vi "Is OD Sub-Entry.vi"(8 "error in":errorcluster, 11 "Section Name in":refnum<class "Section Name.lvclass">) -> (0 "error out":errorcluster, 1 "Is OD Entry?":bool, 2 "Index":u16 format="%.0x", 3 "Section Name out":refnum<class "Section Name.lvclass">)   [LabVIEW 2020, in "Electronic Datasheet.lvlib" / "Section Name.lvclass"]
uses:
  Section Name.lvclass
  Section Name.lvclass/Section Name.ctl
  <vilib>/regexp/Match Regular Expression.xnode
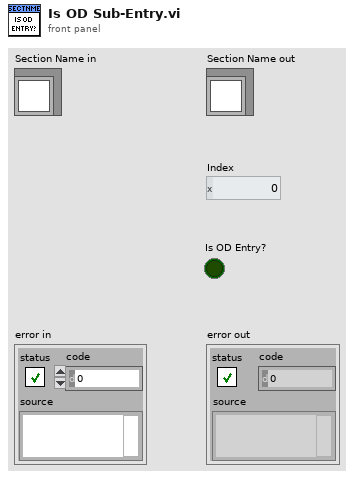
[diagram p1: front panel]
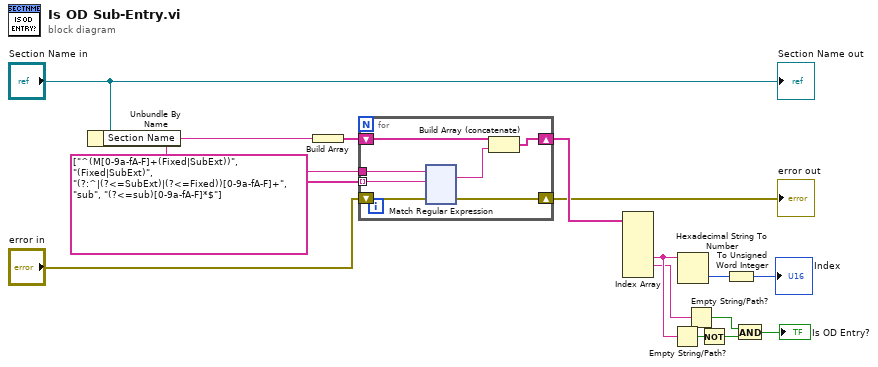
[diagram p0: block diagram]
diagram:
  n1 = Unbundle By Name("Section Name in") -> ("Section Name"=w1:string)
  n2 = Build Array(w1) -> (w14:string[])
  n3 = for {
    tunnel: string[] ["^(M[0-9a-fA-F]+(Fixed|SubExt))", "(Fixed|SubExt)", "(?:^|(?<=SubExt)|(?<=Fixed))[0-9a-fA-F]+", "sub", "(?<=sub)[0-9a-fA-F]*$"] -> [w22] mode=indexing
    shift-right: [w20] -> w12
    shift-left: w14 -> [w21]
    tunnel: w1 -> [w18]
    shift-right: [w16] -> w3
    shift-left: "error in" -> [w17]
    n4 = xnode "Match Regular Expression"("input string"=w18, "regular expression"=w22, "error in"=w17) -> ("whole match"=w19:string, "error out"=w16:errorcluster)  [unwired: 3 in, 3 out]
    n5 = Build Array (concatenate)(w21, w19) -> (w20:string[])
  }
  "error out" <- w3
  n6 = Index Array(array=w12) -> (element #4=w7:string, element #5=w6:string)  [unwired: 6 in, 4 out]
  n7 = Empty String/Path?(string/path=w7) -> (empty?=w10:bool)
  n8 = Hexadecimal String To Number(string=w7) -> (number=w15:u32)  [unwired: 2 in, 1 out]
  n9 = Empty String/Path?(string/path=w6) -> (empty?=w9:bool)
  n10 = Not(x=w10) -> (.not. x?=w5:bool)
  n11 = To Unsigned Word Integer(number=w15) -> (unsigned 16bit integer=→"Index":u16)
  n12 = And(x=w9, y=w5) -> (x .and. y?=→"Is OD Entry?":bool)
  "Section Name out" <- "Section Name in"
